vi "NXT_MIDBRAIN Arbiter.vi"(1 "_irServoCommand":i8, 2 "Behavior Data":T2=[{"Goodness"=[0, 0, 0, 0, 0, 0, 0, 0, 0, 0, 0, 0, 0, 0, 0], "Velocity"=[0, 0, 0, 0, 0, 0, 0, 0, 0, 0, 0, 0, 0, 0, 0], "Weight"=0}, {"Goodness"=[0, 0, 0, 0, 0, 0, 0, 0, 0, 0, 0, 0, 0, 0, 0], "Velocity"=[0, 0, 0, 0, 0, 0, 0, 0, 0, 0, 0, 0, 0, 0, 0], "Weight"=0}, {"Goodness"=[0, 0, 0, 0, 0, 0, 0, 0, 0, 0, 0, 0, 0, 0, 0], "Velocity"=[0, 0, 0, 0, 0, 0, 0, 0, 0, 0, 0, 0, 0, 0, 0], "Weight"=0}], 3 "_motorCommands":T1={"_rudderCommand"=7, "_propCommand"=7, "_irServoCommand"=7}) -> (0 "_motorCommands":T1={"_rudderCommand"=7, "_propCommand"=7, "_irServoCommand"=7})   [LabVIEW 2012, in "Tugboat.lvrbt"]
uses:
  Tugboat.lvrbt
  behaviorData_t.ctl
  behaviorOutput_t.ctl
  motorCommands_t.ctl
panel:
  out "Heading":i8
  out "Speed":i8
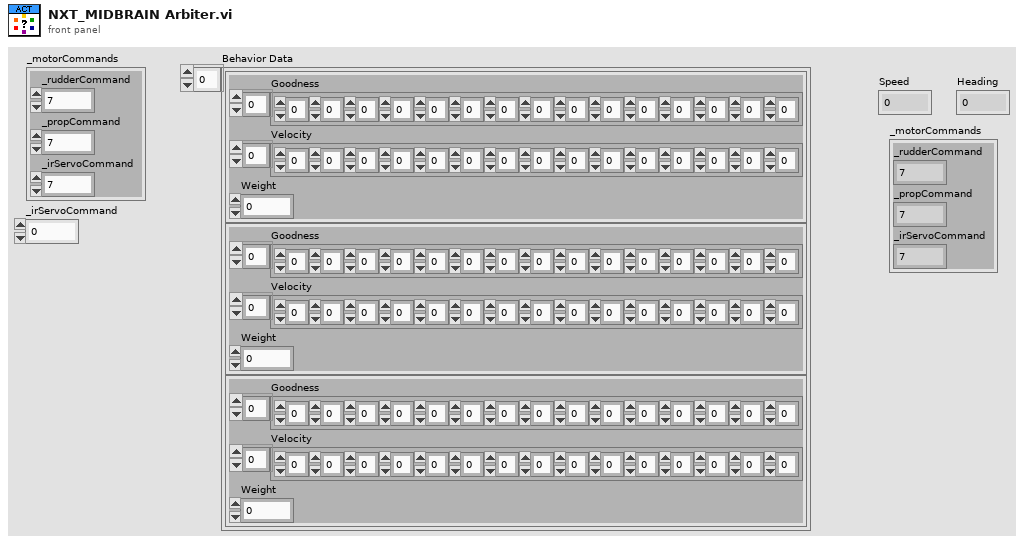
[diagram p1: front panel]
types:
  T1 = typedef "motorCommands_t.ctl" = cluster{"_rudderCommand":i8, "_propCommand":i8, "_irServoCommand":i8}
  T2 = typedef "behaviorData_t.ctl" = T3[]
  T3 = typedef "behaviorOutput_t.ctl" = cluster{"Goodness":i8[], "Velocity":i8[], "Weight":i8}
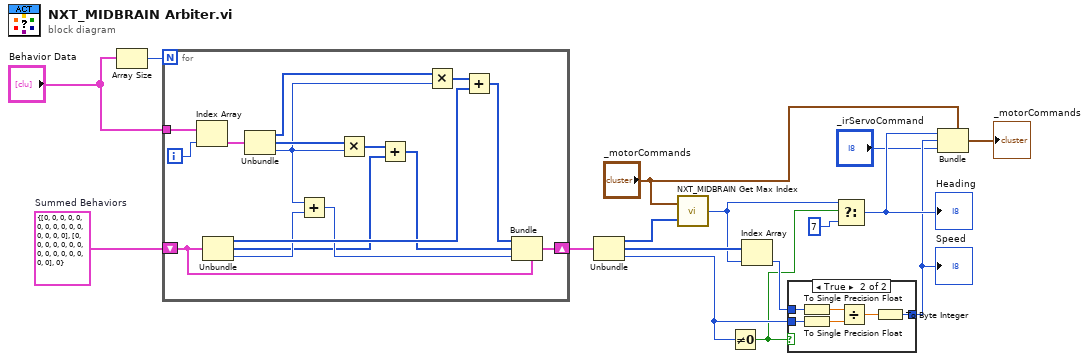
[diagram p0: block diagram]
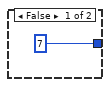
[diagram p2: hidden frame]
diagram:
  w15 = T3 {"Goodness"=[0, 0, 0, 0, 0, 0, 0, 0, 0, 0, 0, 0, 0, 0, 0], "Velocity"=[0, 0, 0, 0, 0, 0, 0, 0, 0, 0, 0, 0, 0, 0, 0], "Weight"=0}  # Summed Behaviors
  n1 = Array Size(array="Behavior Data") -> (size(s)=w16:i32)
  n2 = for {
    N: w16 -> [_]
    shift-right: [w27] -> w13
    shift-left: w15 -> [w28]
    tunnel: "Behavior Data" -> [w31]
    i -> [w32]
    n3 = Index Array(array=w31, index=w32) -> (element=w30:T3)
    n4 = Unbundle(w28) -> ("Goodness"=w25:i8[], "Velocity"=w18:i8[], "Weight"=w23:i8)
    n5 = Unbundle(w30) -> ("Goodness"=w29:i8[], "Velocity"=w21:i8[], "Weight"=w20:i8)
    n6 = Add(x=w20, y=w23) -> (x+y=w22:i8)
    n7 = Multiply(x=w21, y=w20) -> (x*y=w19:i8[])
    n8 = Add(x=w19, y=w18) -> (x+y=w17:i8[])
    n9 = Multiply(x=w29, y=w20) -> (x*y=w26:i8[])
    n10 = Add(x=w26, y=w25) -> (x+y=w24:i8[])
    n11 = Bundle(cluster=w28, "Goodness"=w24, "Velocity"=w17, "Weight"=w22) -> (w27:T3)
  }
  n12 = Unbundle(w13) -> ("Goodness"=w12:i8[], "Velocity"=w11:i8[], "Weight"=w7:i8)
  n13 = call "NXT_MIDBRAIN Get Max Index.vi"("Array"=w12, "_motorCommands"="_motorCommands") -> ("Max Index"=w5:i8)
  n14 = Not Equal To 0?(x=w7) -> (x != 0?=w2:bool)
  n15 = Index Array(array=w11, index=w5) -> (element=w10:i8)
  n16 = case shown="True" w2 {
    tunnel: w10 -> [_ w38]
    tunnel: w7 -> [_ w35]
    tunnel: [i8 7 ("f") w34] -> w3
    frame False {
    }
    frame True {
      n17 = To Single Precision Float(number=w38) -> (single precision float=w39:sgl)
      n18 = To Single Precision Float(number=w35) -> (single precision float=w37:sgl)
      n19 = Divide(x=w39, y=w37) -> (x/y=w36:sgl)
      n20 = To Byte Integer(number=w36) -> (8bit integer=w34:i8)
    }
  }
  "Speed" <- w3
  n21 = Select(t=w5, s=w2, f=i8 7) -> (s? t:f=w6:i8)
  "Heading" <- w6
  n22 = Bundle(cluster="_motorCommands", "_rudderCommand"=w6, "_propCommand"=w3, "_irServoCommand"="_irServoCommand") -> (→"_motorCommands":T1)
